vi "robo_getOpc.vi"(0 "VISA资源名称":refnum<visa-resource-name>, 1 "错误输入（无错误）":errorcluster) -> (2 "VISA资源名称输出":refnum<visa-resource-name>, 3 "数字":i32, 4 "错误输出":errorcluster)   [LabVIEW 2017]
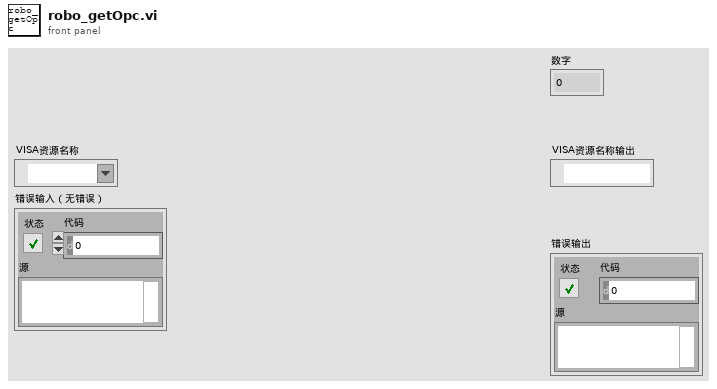
[diagram p1: front panel]
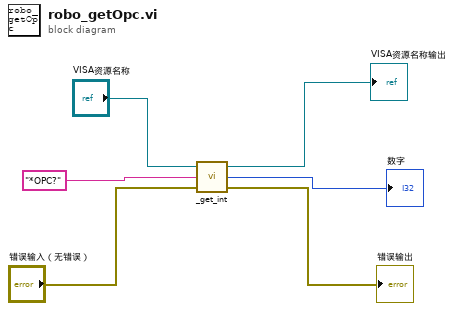
[diagram p0: block diagram]
diagram:
  n1 = call "_get_int.vi"("错误输入（无错误）"="错误输入（无错误）", "写入缓冲区"="*OPC?", "VISA资源名称"="VISA资源名称") -> ("错误输出"=→"错误输出":errorcluster, "数字"=→"数字":i32, "VISA资源名称输出"=→"VISA资源名称输出":refnum<visa-resource-name>)
